vi "Read SysMsg.vi"(8 "error in (no error)":errorcluster, 11 "xData in":refnum<class "xData.lvclass">) -> (0 "error out":errorcluster, 2 "SysMsg":string[](array[string]), 3 "xData out":refnum<class "xData.lvclass">)   [LabVIEW 2014, in "xData.lvclass"]
uses:
  xData.lvclass
  xData.lvclass/xData.ctl
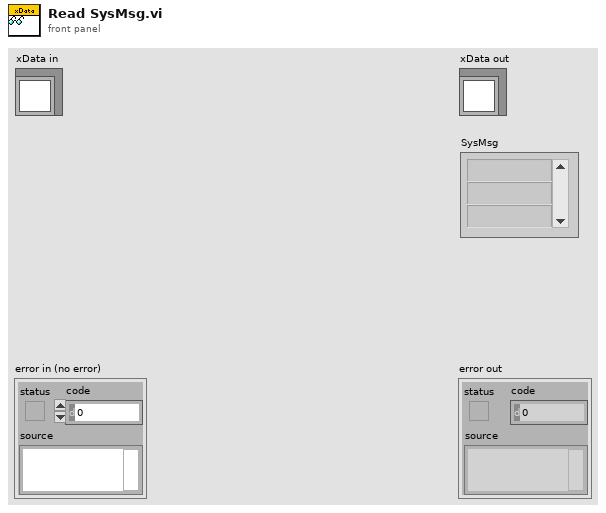
[diagram p1: front panel]
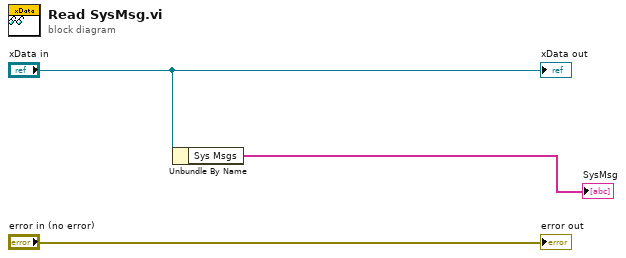
[diagram p0: block diagram]
diagram:
  n1 = Unbundle By Name("xData in") -> ("Sys Msgs"=→"SysMsg":string[])
  "error out" <- "error in (no error)"
  "xData out" <- "xData in"
